vi "ConvertOutputChannelToCommand.vi"(11 "Output Channel (1 or 2)":u8=1 min=1 max=2 step=1) -> (3 "Command":string)   [LabVIEW 2014, in "Keithley-6482-Visa.lvlib"]
uses:
  Keithley-6482-Visa.lvlib
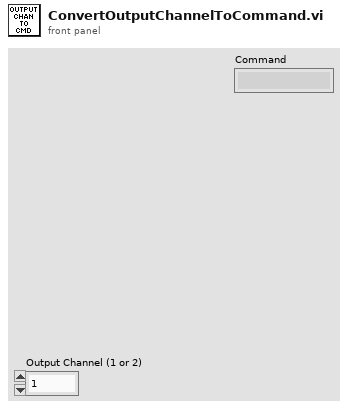
[diagram p1: front panel]
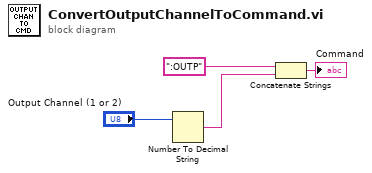
[diagram p0: block diagram]
diagram:
  n1 = Number To Decimal String(number="Output Channel (1 or 2)") -> (decimal integer string=w2:string)  [unwired: 1 in]
  n2 = Concatenate Strings(":OUTP", w2) -> (→"Command":string)
